vi "Split_string_delim.vi"(7 "Ignore case (TRUE def)":bool=TRUE, 10 "Delimiter":string="\\", 11 "Input String":string="c:\\DATA\\20141011-102717-0.fits") -> (1 "Array Length":i32=2, 2 "Conv to number":dbl[](array[numeric]), 3 "Substrings":string[](array[string]), 4 "Strings positions":i32[](array[numeric])=[2, 4], 5 "Empty?":bool)   [LabVIEW 2012]
panel:
  out "indice":i32[](array[numeric])
  out "after substring":string
  out "before substring":string
  out "String Array Selected -- untested":string[](array[string])=["c:\\DATA\\20141011-102717-0.fits", "c:\\DATA\\20141011-102717-1.fits"]
  out "Substrings -- untested - decremented":string[](array[string])=["DATA\\20141011-102717-0.FITS", "20141011-102717-0.FITS"]
  # "use this output for substrings, the rest are tests"
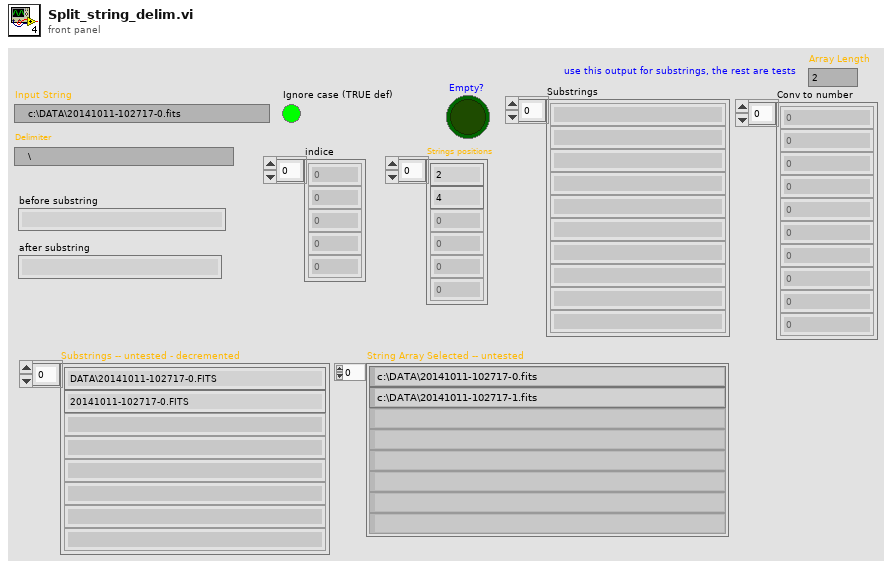
[diagram p1: front panel]
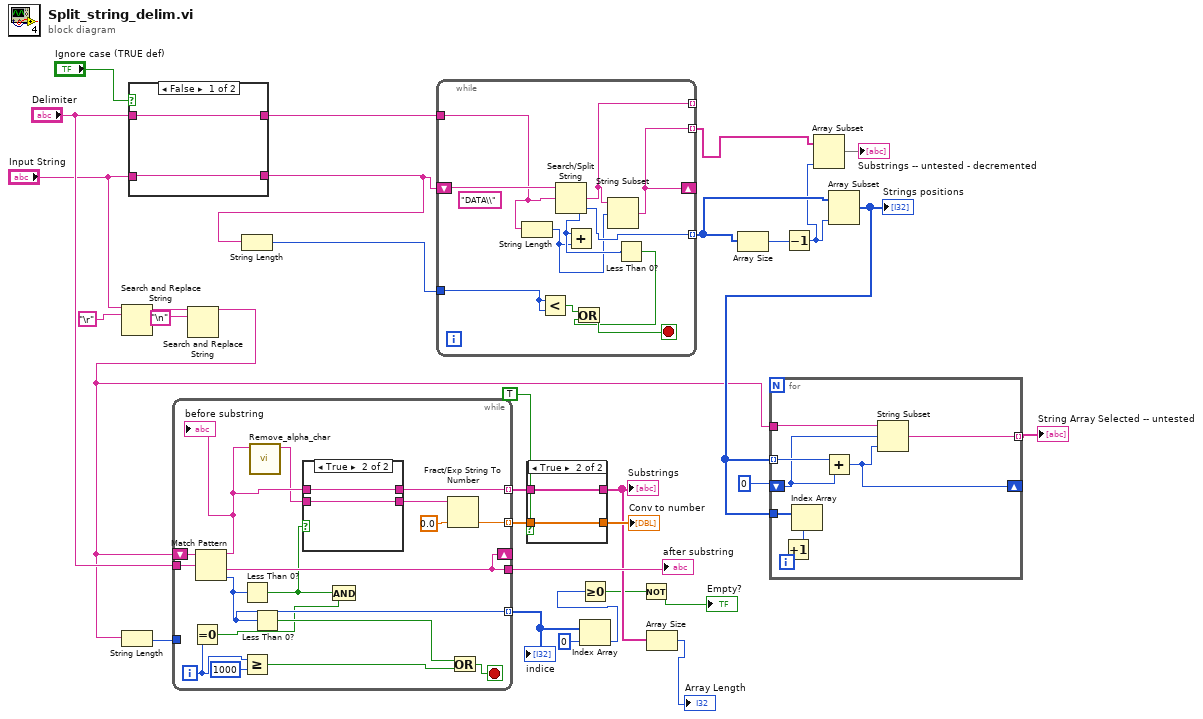
[diagram p0: block diagram]
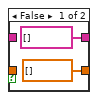
[diagram p2: hidden frame]
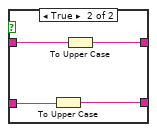
[diagram p4: hidden frame]
diagram:
  n1 = Search and Replace String(input string="Input String", search string="\r") -> (result string=w4:string)  [unwired: 6 in, 3 out]
  n2 = case shown="False" "Ignore case (TRUE def)" {
    tunnel: [w32 w37] -> w31
    tunnel: "Input String" -> [w32 w36]
    tunnel: "Delimiter" -> [w33 w35]
    tunnel: [w33 w34] -> w28
    frame False {
    }
    frame True {
      n3 = To Upper Case(1:w36) -> (0:w37:string)
      n4 = To Upper Case(1:w35) -> (0:w34:string)
    }
  }
  n5 = Search and Replace String(input string=w4, search string="\n") -> (result string=w2:string)  [unwired: 6 in, 3 out]
  n6 = String Length(string=w2) -> (length=w17:i32)
  n7 = while {
    tunnel: [w41] -> w13 mode=indexing
    tunnel: [w47] -> w19
    tunnel: "Delimiter" -> [w54]
    shift-right: [w47] -> _
    shift-left: w2 -> [w53]
    tunnel: [w45] -> w16 mode=indexing
    tunnel: w17 -> [_]
    tunnel: [w46] -> w12 mode=indexing
    i -> [w44]
    stop <- w51 stop-if-true
    n8 = Equal To 0?(x=w44) -> (x = 0?=w43:bool)
    n9 = Match Pattern(string=w53, regular expression=w54) -> (before substring=w42:string, after substring=w47:string, offset past match=w45:i32)  [unwired: 1 in, 1 out]
    "before substring" <- w42
    n10 = Less Than 0?(x=w45) -> (x < 0?=w38:bool)
    n11 = Greater Or Equal?(x=w44, y=1000) -> (x >= y?=w52:bool)
    n12 = call "Remove_alpha_char.vi"("input string"=w42) -> ("Result"=w40:string)  [unwired: 10 in]
    n13 = Less Than 0?(x=w45) -> (x < 0?=w48:bool)
    n14 = case shown="True" w38 {
      tunnel: w42 -> [w56 w58]
      tunnel: [w56 w58] -> w41
      tunnel: w40 -> [w55 w57]
      tunnel: [w55 w57] -> w39
      frame False {
      }
      frame True {
      }
    }
    n15 = And(x=w38, y=w43) -> ()  [unwired: 1 out]
    n16 = Fract/Exp String To Number(string=w39, default (0 dbl)=0.0 ("default (0 I32)")) -> (number=w46:dbl)  [unwired: 2 in, 1 out]
    n17 = Or(x=w48, y=w52) -> (x .or. y?=w51:bool)
  }
  "after substring" <- w19
  "indice" <- w16
  n18 = String Length(string=w31) -> (length=w30:i32)
  n19 = while {
    shift-right: [w65] -> _
    shift-left: w31 -> [w66]
    tunnel: [w65] -> w27 mode=indexing
    tunnel: w30 -> [w63]
    tunnel: [w62] -> w25 mode=indexing
    tunnel: [w60] -> _ mode=indexing
    tunnel: w28 -> [w59]
    stop <- w67 stop-if-true
    (unwired) "DATA\\" ("search string/char (-)")
    n20 = String Length(string=w59) -> (length=w61:i32)
    n21 = Less?(x=w63, y=w63) -> (x < y?=w68:bool)
    n22 = Search/Split String(string=w66, search string/char (-)=w59) -> (match + rest of string=w60:string, offset of match=w62:i32)  [unwired: 1 in, 1 out]
    n23 = Add(x=w62, y=w61) -> ()  [unwired: 1 out]
    n24 = String Subset(string=w60, offset (0)=w61) -> (substring=w65:string)  [unwired: 1 in]
    n25 = Less Than 0?(x=w62) -> (x < 0?=w64:bool)
    n26 = Or(x=w68, y=w64) -> (x .or. y?=w67:bool)
  }
  n27 = case shown="True" TRUE {
    tunnel: w13 -> [_ w72]
    tunnel: [string[] [] w72] -> w10
    tunnel: w12 -> [_ w71]
    tunnel: [dbl[] [] w71] -> w11
    frame False {
    }
    frame True {
    }
  }
  "Substrings" <- w10
  "Conv to number" <- w11
  n28 = Index Array(array=w16, index=0) -> (element=w14:i32)
  n29 = Greater Or Equal To 0?(x=w14) -> (x >= 0?=w8:bool)
  n30 = Not(x=w8) -> (.not. x?=→"Empty?":bool)
  n31 = Array Size(array=w10) -> (size(s)=→"Array Length":i32)
  n32 = Array Size(array=w25) -> (size(s)=w26:i32)
  n33 = Decrement(x=w26) -> (x-1=w20:i32)
  n34 = Array Subset(array=w27, length=w20) -> (→"Substrings -- untested - decremented":string[])  [unwired: 1 in]
  n35 = Array Subset(array=w25, length=w20) -> (w22:i32[])  [unwired: 1 in]
  "Strings positions" <- w22
  n36 = for {
    tunnel: w2 -> [w80]
    tunnel: w22 -> [w79] mode=indexing
    shift-right: [w74] -> _
    shift-left: 0 -> [w73]
    tunnel: w22 -> [w77]
    tunnel: [w75] -> w21 mode=indexing
    i -> [w78]
    n37 = Increment(x=w78) -> (x+1=w76:i32)
    n38 = Index Array(array=w77, index=w76) -> ()  [unwired: 1 out]
    n39 = Add(x=w79, y=w73) -> (x+y=w74:i32)
    n40 = String Subset(string=w80, offset (0)=w73, length (rest)=w74) -> (substring=w75:string)
  }
  "String Array Selected -- untested" <- w21
